vi "sv_Compute Recursive Filter Coefficients.vi"(6 "model":i32(ring) items=["Absolute acceleration", "Relative displacement"], 9 "dt [s]":dbl=2e-05 format="%.2e", 10 "critical damping factor":dbl=0.05 format="%.2f", 11 "fn [Hz]":dbl=100.0 format="%.2f") -> (2 "forward coefficients":dbl[](array[numeric]) format="%.2e", 3 "reverse coefficients":dbl[](array[numeric]) format="%.2e")   [LabVIEW 2017, in "SoundVib_Transient.lvlib"]
uses:
  <vilib>/addons/Sound and Vibration/svt_Transients/SoundVib_Transient.lvlib
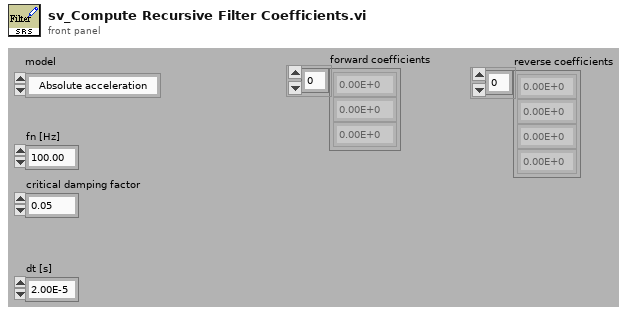
[diagram p1: front panel]
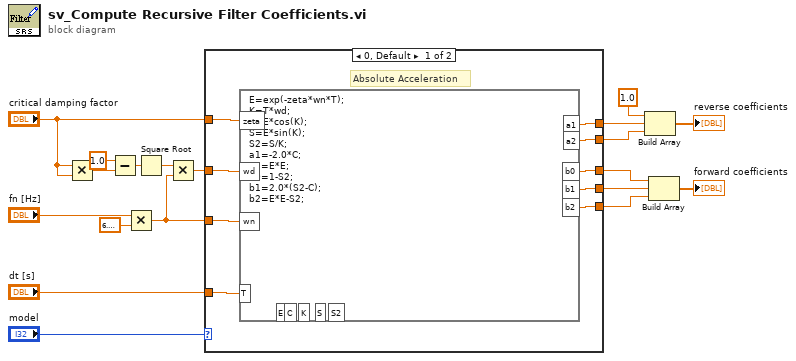
[diagram p0: block diagram]
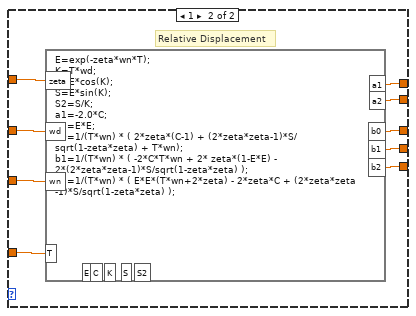
[diagram p2: hidden frame]
diagram:
  n1 = Multiply(x="critical damping factor", y="critical damping factor") -> (x*y=w3:dbl)
  n2 = Subtract(x=1.0, y=w3) -> (x-y=w4:dbl)
  n3 = Multiply(x="fn [Hz]", y=6.283185307179586) -> (x*y=w16:dbl)
  n4 = Square Root(x=w4) -> (sqrt(x)=w1:dbl)
  n5 = Multiply(x=w1, y=w16) -> (x*y=w17:dbl)
  n6 = case shown="0, Default" "model" {
    tunnel: w17 -> [w27 w37]
    tunnel: w16 -> [w26 w36]
    tunnel: "dt [s]" -> [w25 w35]
    tunnel: "critical damping factor" -> [w28 w34]
    tunnel: [w23 w33] -> w14
    tunnel: [w24 w32] -> w13
    tunnel: [w21 w31] -> w12
    tunnel: [w20 w30] -> w11
    tunnel: [w22 w29] -> w10
    frame 0, Default {
      # "Absolute Acceleration"
      n7 = formula code="E=exp(-zeta*wn*T);\nK=T*wd;\nC=E*cos(K);\nS=E*sin(K);\nS2=S/K;\na1=-2.0*C;\na2=E*E;\nb0=1-S2;\nb1=2.0*(S2-C);\nb2=E*E-S2;"("wd"=w27, "wn"=w26, "T"=w25, "zeta"=w28) -> ("a1"=w24:dbl, "a2"=w23:dbl, "b1"=w21:dbl, "b2"=w20:dbl, "b0"=w22:dbl)  [unwired: 5 out]
    }
    frame 1 {
      # "Relative Displacement"
      n8 = formula code="E=exp(-zeta*wn*T);\nK=T*wd;\nC=E*cos(K);\nS=E*sin(K);\nS2=S/K;\na1=-2.0*C;\na2=E*E;\nb0=1/(T*wn) * ( 2*zeta*(C-1) + (2*zeta*zeta-1)*S/sqrt(1-zeta*zeta) + T*wn);\nb1=1/(T*wn) * ( -2*C*T*wn + 2* zeta*(1-E*E) - 2*(2*zeta*zeta-1)*S/sqrt(1-zeta*zeta) );\nb2=1/(T*wn) * ( E*E*(T*wn+2*zeta) - 2*zeta*C + (2*zeta*zeta -1)*S/sqrt(1-zeta*zeta) );"("wd"=w37, "wn"=w36, "T"=w35, "zeta"=w34) -> ("a1"=w32:dbl, "a2"=w33:dbl, "b1"=w31:dbl, "b2"=w30:dbl, "b0"=w29:dbl)  [unwired: 5 out]
    }
  }
  n9 = Build Array(1.0, w13, w14) -> (→"reverse coefficients":dbl[])
  n10 = Build Array(w10, w12, w11) -> (→"forward coefficients":dbl[])
